vi "sub parse frame basic.vi"(8 "error in (no error)":errorcluster, 11 "String":string="   pic 7 state 1 wait 3 next 999 centerx 48 centery 83 hit_Fa 285 hit_Fj 273 hit_Uj 250 hit_Dj 260 hit_ja 295") -> (0 "error out":errorcluster, 3 "frame basic data":T1)   [LabVIEW 2018, in "Frame Analizer.lvclass"]
uses:
  Frame Analizer.lvclass
  frame basic data.ctl
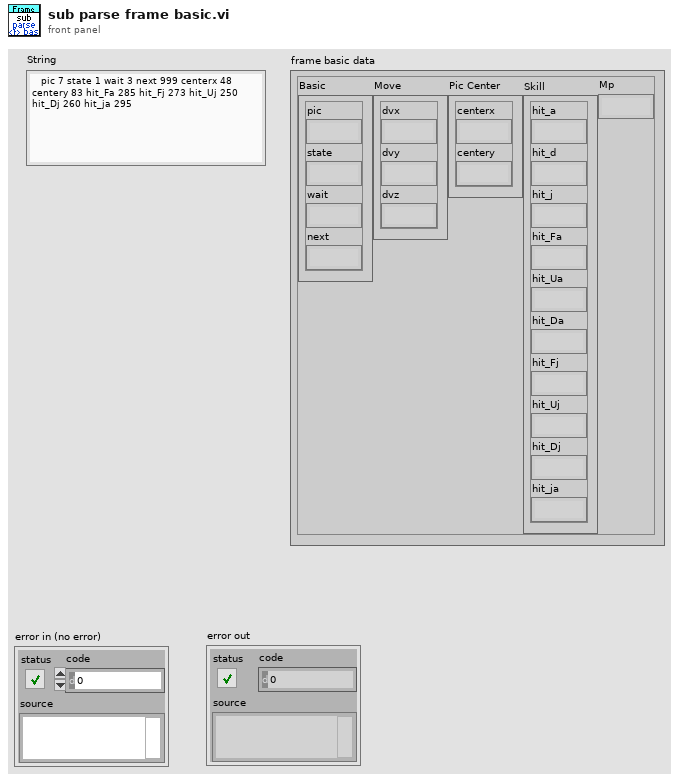
[diagram p1: front panel]
types:
  T1 = typedef "Frame Analizer.lvclass/frame basic data.ctl" = cluster{"Basic":cluster{"pic":string, "state":string, "wait":string, "next":string}, "Move":cluster{"dvx":string, "dvy":string, "dvz":string}, "Pic Center":cluster{"centerx":string, "centery":string}, "Skill":cluster{"hit_a":string, "hit_d":string, "hit_j":string, "hit_Fa":string, "hit_Ua":string, "hit_Da":string, "hit_Fj":string, "hit_Uj":string, "hit_Dj":string, "hit_ja":string}, "Mp":string}
  T2 = cluster{"[0]":string, "[1]":string, "[2]":string, "[3]":string}
  T3 = cluster{"[0]":string, "[1]":string, "[2]":string}
  T4 = cluster{"[0]":string, "[1]":string, "[2]":string, "[3]":string, "[4]":string, "[5]":string, "[6]":string, "[7]":string, "[8]":string, "[9]":string}
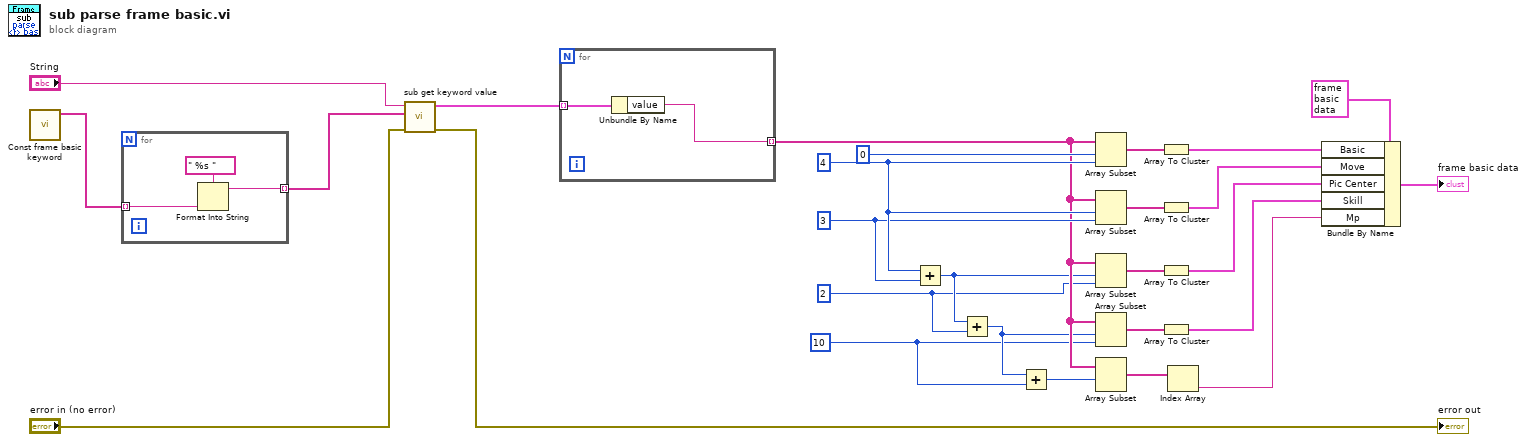
[diagram p0: block diagram]
diagram:
  w11 = 10 ("length")
  w13 = 2 ("length")
  w23 = 3 ("length")
  w24 = 4 ("length")
  n1 = call "Const frame basic keyword.vi"() -> ("Const frame basic keyword"=w2:string[])  [unwired: 11 in]
  n2 = for {
    tunnel: w2 -> [w30] mode=indexing
    tunnel: [w28] -> w1 mode=indexing
    n3 = Format Into String(format string=" %s ", w30) -> (resulting string=w28:string)  [unwired: 2 in, 1 out]
  }
  n4 = call "sub get keyword value.vi"("error in"="error in (no error)", "keyword"=w1, "string"="String") -> ("error out"=→"error out":errorcluster, "matched pairs (all)"=w26:cluster{"keyword":string, "value":string}[])  [unwired: 5 in, 2 out]
  n5 = for {
    tunnel: w26 -> [w32] mode=indexing
    tunnel: [w31] -> w15 mode=indexing
    n6 = Unbundle By Name(w32) -> ("value"=w31:string)
  }
  n7 = Add(x=w24, y=w23) -> (x+y=w14:i32)
  n8 = Add(x=w14, y=w13) -> (x+y=w12:i32)
  n9 = Add(x=w12, y=w11) -> (x+y=w22:i32)
  n10 = Array Subset(array=w15, index=0, length=w24) -> (w21:string[])
  n11 = Array Subset(array=w15, index=w24, length=w23) -> (w20:string[])
  n12 = Array Subset(array=w15, index=w14, length=w13) -> (w19:string[])
  n13 = Array Subset(array=w15, index=w12, length=w11) -> (w6:string[])
  n14 = Array Subset(array=w15, index=w22) -> (w4:string[])  [unwired: 1 in]
  n15 = Array To Cluster(array=w21) -> (cluster=w18:T2)
  n16 = Array To Cluster(array=w20) -> (cluster=w17:T3)
  n17 = Array To Cluster(array=w19) -> (cluster=w16:cluster{"[0]":string, "[1]":string})
  n18 = Array To Cluster(array=w6) -> (cluster=w5:T4)
  n19 = Index Array(array=w4) -> (element=w3:string)  [unwired: 1 in]
  n20 = Bundle By Name(cluster=T1 {"Basic"={"pic"="176", "state"="3", "wait"="1", "next"="287"}, "Move"={"dvx"="10", "dvy"="", "dvz"="1"}, "Pic Center"={"centerx"="32", "centery"="90"}, "Skill"={"hit_a"="", "hit_d"="288", "hit_j"="288", "hit_Fa"="", "hit_Ua"="", "hit_Da"="", "hit_Fj"="", "hit_Uj"="", "hit_Dj"="", "hit_ja"=""}, "Mp"="-17"} ("frame basic data 2"), "Basic"=w18, "Move"=w17, "Pic Center"=w16, "Skill"=w5, "Mp"=w3) -> (→"frame basic data":T1)
